vi "Queue Manager.vi"(6 "Action (Back)":enum16{"Back", "Front", "Replace"}(ring), 8 "error in (no error)":errorcluster, 10 "Elements":cluster{"State":T1, "Data":variant}[](array[cluster]), 11 "Queue In":refnum<queue>) -> (0 "error out":errorcluster, 3 "Queue Out":refnum<queue>)   [LabVIEW 2013, in "VI Internal QSM.lvlib"]
uses:
  VI Internal QSM.lvlib
  UserDefined Control/QSM State.ctl
  UserDefined Control/QSM Msg.ctl
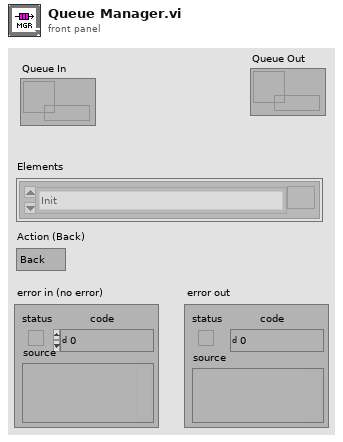
[diagram p1: front panel]
types:
  T1 = typedef "VI Internal QSM.lvlib/QSM State.ctl" = enum16{"Init", "Idle", "Error", "Exit", "Test"}
  T2 = typedef "VI Internal QSM.lvlib/QSM Msg.ctl" = cluster{"State":T1, "Data":variant}
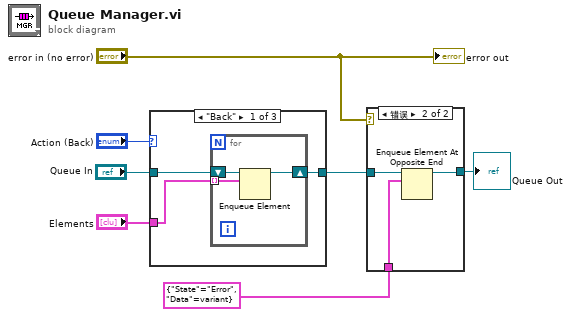
[diagram p0: block diagram]
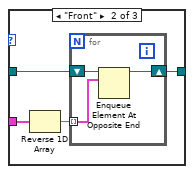
[diagram p3: hidden frame]
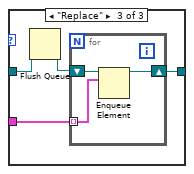
[diagram p4: hidden frame]
diagram:
  n1 = case shown="\"Back\"" "Action (Back)" {
    tunnel: "Queue In" -> [w10 w17 w22]
    tunnel: "Elements" -> [w9 w16 w23]
    tunnel: [w8 w15 w24] -> w5
    frame "Back" {
      n2 = for {
        tunnel: w9 -> [w12] mode=indexing
        shift-right: [w11] -> w8
        shift-left: w10 -> [w13]
        n3 = Enqueue Element(queue=w13, element=w12) -> (queue out=w11:refnum<queue>)  [unwired: 1 in, 3 out]
      }
    }
    frame "Front" {
      n4 = Reverse 1D Array(array=w16) -> (reversed array=w14:cluster{"State":T1, "Data":variant}[])
      n5 = for {
        tunnel: w14 -> [w19] mode=indexing
        shift-right: [w18] -> w15
        shift-left: w17 -> [w20]
        n6 = Enqueue Element At Opposite End(queue=w20, element=w19) -> (queue out=w18:refnum<queue>)  [unwired: 1 in, 3 out]
      }
    }
    frame "Replace" {
      n7 = Flush Queue(queue=w22) -> (queue out=w21:refnum<queue>)  [unwired: 1 in, 2 out]
      n8 = for {
        tunnel: w23 -> [w26] mode=indexing
        shift-right: [w25] -> w24
        shift-left: w21 -> [w27]
        n9 = Enqueue Element(queue=w27, element=w26) -> (queue out=w25:refnum<queue>)  [unwired: 1 in, 3 out]
      }
    }
  }
  n10 = case shown="错误" "error in (no error)" {
    tunnel: w5 -> [w28 w31]
    tunnel: T2 {"State"=enum."Error", "Data"=variant} ("Msg") -> [_ w30]
    tunnel: [w28 w29] -> w2
    frame No Error {
    }
    frame Error {
      n11 = Enqueue Element At Opposite End(queue=w31, element=w30) -> (queue out=w29:refnum<queue>)  [unwired: 1 in, 3 out]
    }
  }
  "Queue Out" <- w2
  "error out" <- "error in (no error)"
